vi "remove tag.vi"(8 "error in":errorcluster, 10 "tag":refnum<class "tag descriptor.lvclass">, 11 "tag collection in":refnum<class "tag collection.lvclass">) -> (0 "error out":errorcluster, 1 "removed tag":refnum<class "tag descriptor.lvclass">, 3 "tag collection out":refnum<class "tag collection.lvclass">)   [LabVIEW 2013, in "tag bus.lvlib" / "tag collection.lvclass"]
uses:
  tag collection.lvclass
  tag/tag descriptor.lvclass
  tag collection.lvclass/tag collection.ctl
  tag/tag descriptor.lvclass/tag descriptor.ctl
  tag bus.lvlib
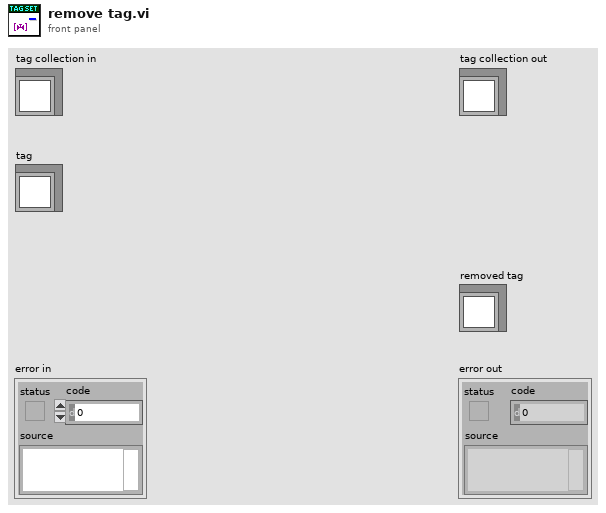
[diagram p1: front panel]
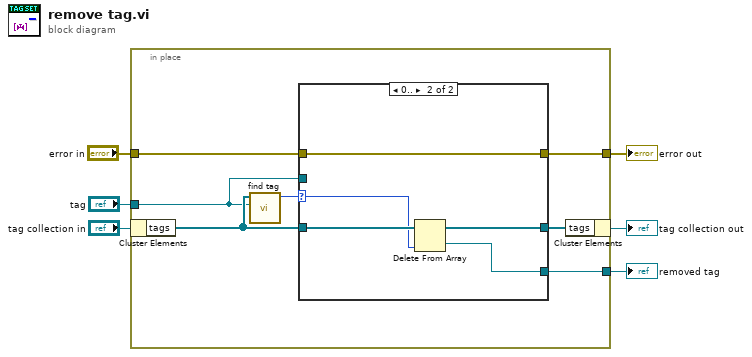
[diagram p0: block diagram]
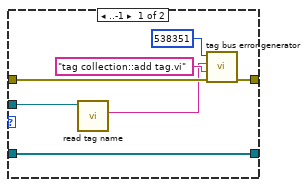
[diagram p2: hidden frame]
diagram:
  n1 = in-place {
    in-place-border: "error in" -> [w12]
    in-place-border: [w13] -> w3
    in-place-border: "tag" -> [w8]
    in-place-border: [w7] -> w1
    n2 = in-place-cluster #1("tag collection in") -> ("tags"=w9:refnum<class "tag descriptor.lvclass">[])
    n3 = call "find tag.vi"("tag"=w8, "tags in"=w9) -> ("index"=w10:i32)  [unwired: 9 in]
    n4 = case shown="0.." w10 {
      selector: w10 -> [_ w22]
      tunnel: [w18 w25] -> w13
      tunnel: w12 -> [w19 w25]
      tunnel: w9 -> [w20 w24]
      tunnel: [w20 w23] -> w11
      tunnel: w8 -> [w15 _]
      tunnel: [_ w21] -> w7
      frame ..-1 {
        n5 = call "read tag name.vi"("system tag in"=w15) -> ("name"=w14:string)  [unwired: 8 in, 2 out]
        n6 = call "tag bus error generator.vi"("error in"=w19, "source"="tag collection::add tag.vi", "append error message"=w14, "error code (0)"=538351) -> ("error out"=w18:errorcluster)  [unwired: 5 in]
      }
      frame 0.. {
        n7 = Delete From Array(array=w24, index=w22) -> (deleted portion=w21:refnum<class "tag descriptor.lvclass">, array with subset deleted=w23:refnum<class "tag descriptor.lvclass">[])  [unwired: 1 in]
      }
    }
    n8 = in-place-cluster #1("tags"=w11) -> (→"tag collection out":refnum<class "tag collection.lvclass">)
  }
  "error out" <- w3
  "removed tag" <- w1
